vi "MC.DangwooOptron.SetResource.vi"(8 "error in (no error)":errorcluster, 10 "Resource":T1, 11 "MC.DangwooOptron":refnum<class "MC.DangwooOptron.lvclass">) -> (0 "error out":errorcluster, 3 "MC.DangwooOptron out":refnum<class "MC.DangwooOptron.lvclass">)   [LabVIEW 2017, in "MC.DangwooOptron.lvclass"]
doc: "JKI State Machine Objects (SMO) 1.0.0.5\nJKI - JKI\nCopyright (c) 2016, JKI"
uses:
  MC.DangwooOptron.lvclass
  Typedefs/Resource--Cluster.ctl
  MC.DangwooOptron.lvclass/MC.DangwooOptron.ctl
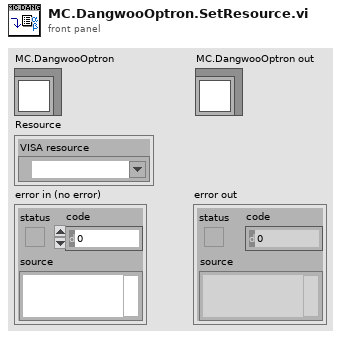
[diagram p1: front panel]
types:
  T1 = typedef "MC.DangwooOptron.lvclass/Resource--Cluster.ctl" = cluster{"VISA resource":refnum<visa-resource-name>}
  T2 = typedef "MC.DangwooOptron.lvclass/PrivateData--Ref.ctl" = refnum<data-value>
  T3 = typedef "MC.DangwooOptron.lvclass/PrivateData--Cluster.ctl" = cluster{"Resource":T1}
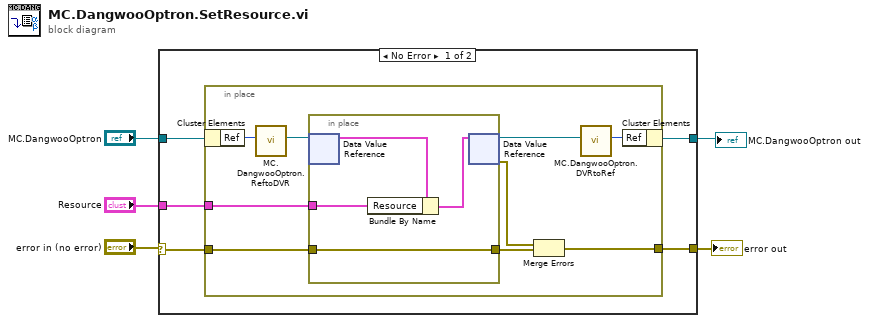
[diagram p0: block diagram]
diagram:
  n1 = case shown="No Error" "error in (no error)" {
    selector: "error in (no error)" -> [w8 w24]
    tunnel: [w10 w25] -> w5
    tunnel: "MC.DangwooOptron" -> [w9 w25]
    tunnel: "Resource" -> [w7 _]
    tunnel: [w6 w24] -> w1
    frame No Error {
      n2 = in-place {
        in-place-border: w8 -> [w16]
        in-place-border: w7 -> [w15]
        in-place-border: [w11] -> w6
        n3 = in-place-cluster #1(w9) -> ("Ref"=w19:u32)
        n4 = call "MC.DangwooOptron.ReftoDVR.vi"("Ref"=w19) -> ("Ref"=w18:T2)  [unwired: 10 in]
        n5 = in-place {
          in-place-border: w16 -> [w20]
          in-place-border: w15 -> [w21]
          in-place-border: [w20] -> w13
          n6 = in-place-dvr #2(w18) -> (w23:T3)  [unwired: 1 out]
          n7 = Bundle By Name(cluster=w23, "Resource"=w21) -> (w22:T3)
          n8 = in-place-dvr #2(w22) -> (w14:T2, w12:errorcluster)
        }
        n9 = Merge Errors(w12, w13) -> (w11:errorcluster)
        n10 = call "MC.DangwooOptron.DVRtoRef.vi"("Ref"=w14) -> ("Ref"=w17:u32)  [unwired: 10 in]
        n11 = in-place-cluster #1("Ref"=w17) -> (w10:refnum<class "MC.DangwooOptron.lvclass">)
      }
    }
    frame Error {
    }
  }
  "error out" <- w1
  "MC.DangwooOptron out" <- w5
